vi "Read U8.vi"(8 "error in (no error)":errorcluster, 10 "Tag":string, 11 "Var Bus in":refnum<class "Multi_Bus.lvclass">) -> (0 "error out":errorcluster, 2 "Numeric":u8, 3 "Var Bus out":refnum<class "Multi_Bus.lvclass">)   [LabVIEW 2021, in "Multi_Bus.lvclass"]
uses:
  Multi_Bus.lvclass
  Multi_Bus.lvclass/Multi_Bus.ctl
  <vilib>/TSA/Abstract Data Classes/Abs_Types/U8 Integer/Abs_U8 Integer.lvclass
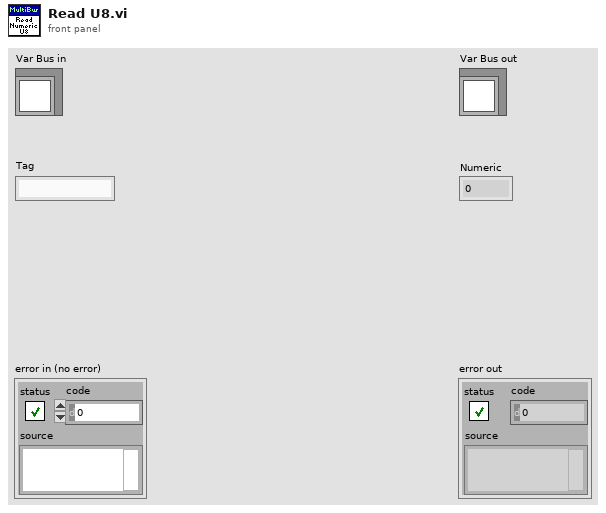
[diagram p1: front panel]
types:
  T1 = typedef "Abs_U8 Integer.lvclass/Type.ctl" = u8
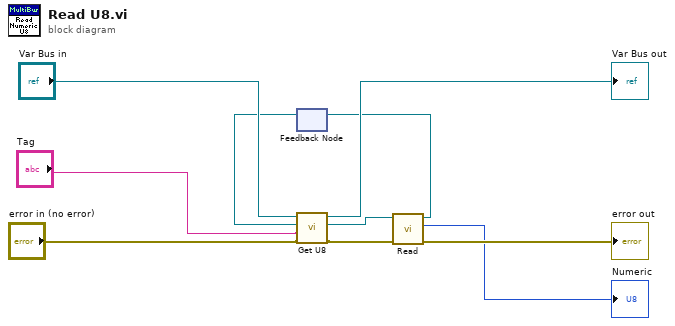
[diagram p0: block diagram]
diagram:
  n1 = feedback #1() -> (w1:refnum<class "Abs_U8 Integer.lvclass">)  [unwired: 1 in]
  n2 = call-dynamic "Get U8.vi"("error in (no error)"="error in (no error)", "Tag"="Tag", "Value Type"=w1, "Var Bus in"="Var Bus in") -> ("error out"=w3:errorcluster, "Value Out"=w2:refnum<class "Abs_U8 Integer.lvclass">, "Var Bus out"=→"Var Bus out":refnum<class "Multi_Bus.lvclass">)  [unwired: 5 in]
  n3 = call-dynamic "Read.vi"("error in (no error)"=w3, "Double Float.lvclass_340760 in"=w2) -> ("error out"=→"error out":errorcluster, "Value"=→"Numeric":T1, "Double Float.lvclass_340760 out"=w4:refnum<class "Abs_U8 Integer.lvclass">)  [unwired: 7 in]
  n4 = feedback-in #1(w4) -> ()
